vi "sample4(SyncRW X).vi"() -> ()   [LabVIEW 2020]
panel:
  in  "OffsetTime":u32=500
  out "SyncRead Data":cluster{"ID":u8, "Error":u16, "RTTick":u16}[](array[cluster]) {"Error" format="%04x"}
  in  "id3":u8=3 max=253
  in  "id2":u8=2 max=253
  in  "id1":u8=1 max=253
  in  "pos3":i32(knob)
  in  "STOP":bool
  in  "pos2":i32(knob)
  in  "pos1":i32(knob)
  in  "COM":refnum<visa-resource-name> caption="COMポート"
  in  "Baudrate":i32=57600
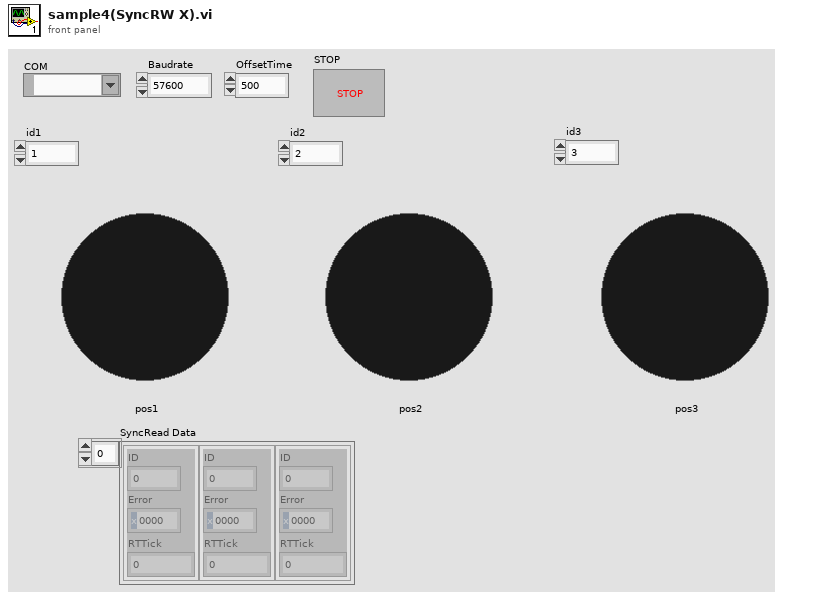
[diagram p1: front panel]
types:
  T1 = cluster{"X Address":u16, "size":u16, cluster{"id3":u8, "array":u8[]}[]}
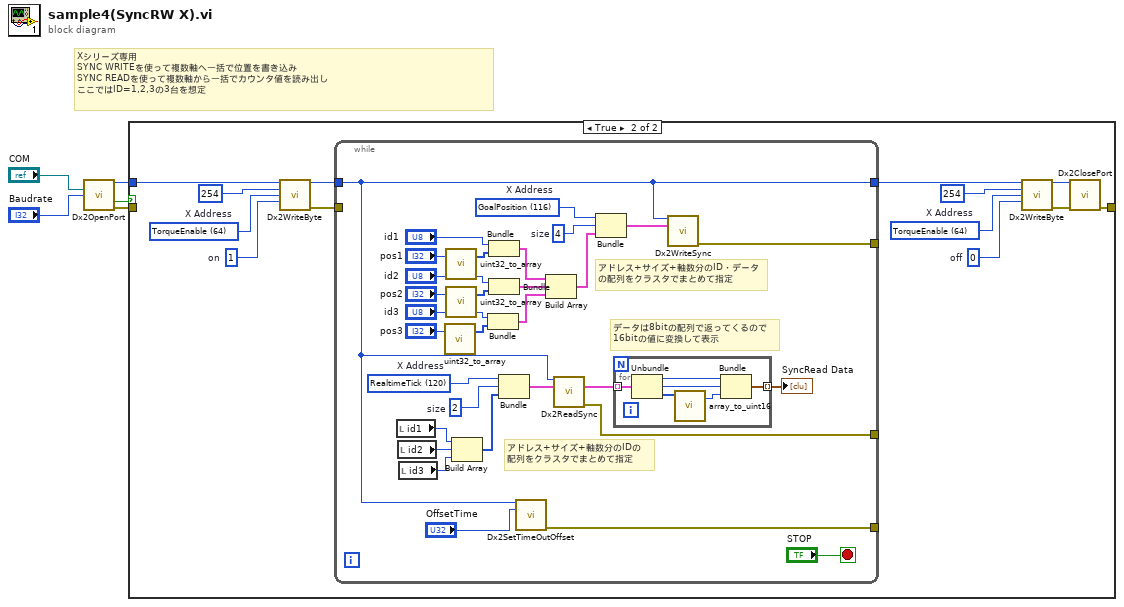
[diagram p0: block diagram]
diagram:
  # "Xシリーズ専用\nSYNC WRITEを使って複数軸へ一括で位置を書き込み\nSYNC READを使って複数軸から一括でカウンタ値を読み出し\nここではID=1,2,3の3台を想定"
  n1 = call "Dx2OpenPort.vi"("port"="COM", "baudrate"="Baudrate") -> ("dvid"=w5:u32, "成功"=w2:bool, "エラー出力"=w1:errorcluster)  [unwired: 11 in]
  n2 = case shown="TRUE" w2 {
    tunnel: w5 -> [_ w17]
    tunnel: w1 -> [_ _]
    tunnel: [_ w13] -> _
    frame False {
    }
    frame True {
      w7 = u16 64 items=["ModelNo"=0, "ModelInfo"=2, "VersionOfFirmware"=6, "ID"=7, "Baudrate"=8, "ReturnDelayTime"=9, "OperationMode"=11, "ProtocolVersion"=13, "HormingOffset"=20, "MovingThreshold"=24, "TemperatureLimit"=31, "MaxVoltageLimit"=32, "MinVoltageLimit"=34, "PWMLimit"=36, "CurrentLimit"=38, "AccelerationLimit"=40, "VelocityLimit"=44, "MaxPositionLimit"=48, "MinPositionLimit"=52, "Shutdown"=63, "TorqueEnable"=64, "LED"=65, "StatusReturnLevel"=68, "RegistedInstruction"=69, "HardwareErrorStatus"=70, "VelocityIGain"=76, "VelocityPGain"=78, "VelocityDGain"=80, "PositionIGain"=82, "PositionPGain"=84, "FeedForward2ndGain"=88, "FeedForward1stGain"=90, "GoalPWM"=100, "GoalCurrent"=102, "GoalVelocity"=104, "ProfileAcceleration"=108, "ProfileVelocity"=112, "GoalPosition"=116, "RealtimeTick"=120, "Moving"=122, "MovingStatus"=123, "PresentPWM"=124, "PresentCurrent"=126, "Presentvelocity"=128, "PresentPosition"=132, "VelocityTrajectory"=136, "PositionTrajectory"=140, "PresentIInputVoltage"=144, "PresentTemperature"=146, "Backup Ready"=147]  # X Address
      w6 = u16 64 items=["ModelNo"=0, "ModelInfo"=2, "VersionOfFirmware"=6, "ID"=7, "Baudrate"=8, "ReturnDelayTime"=9, "OperationMode"=11, "ProtocolVersion"=13, "HormingOffset"=20, "MovingThreshold"=24, "TemperatureLimit"=31, "MaxVoltageLimit"=32, "MinVoltageLimit"=34, "PWMLimit"=36, "CurrentLimit"=38, "AccelerationLimit"=40, "VelocityLimit"=44, "MaxPositionLimit"=48, "MinPositionLimit"=52, "Shutdown"=63, "TorqueEnable"=64, "LED"=65, "StatusReturnLevel"=68, "RegistedInstruction"=69, "HardwareErrorStatus"=70, "VelocityIGain"=76, "VelocityPGain"=78, "VelocityDGain"=80, "PositionIGain"=82, "PositionPGain"=84, "FeedForward2ndGain"=88, "FeedForward1stGain"=90, "GoalPWM"=100, "GoalCurrent"=102, "GoalVelocity"=104, "ProfileAcceleration"=108, "ProfileVelocity"=112, "GoalPosition"=116, "RealtimeTick"=120, "Moving"=122, "MovingStatus"=123, "PresentPWM"=124, "PresentCurrent"=126, "Presentvelocity"=128, "PresentPosition"=132, "VelocityTrajectory"=136, "PositionTrajectory"=140, "PresentIInputVoltage"=144, "PresentTemperature"=146, "Backup Ready"=147]  # X Address
      w11 = u8 0  # off
      w18 = u8 1  # on
      n3 = call "Dx2WriteByte.vi"("dvid in"=w17, "id"=u8 254, "address"=w6, "data in"=w18) -> ("dvid out"=w15:u32, "エラー出力"=w14:errorcluster)  [unwired: 9 in, 1 out]
      n4 = while {
        tunnel: [w48] -> _
        tunnel: [w46] -> _
        tunnel: w15 -> [w23]
        tunnel: w14 -> [_]
        tunnel: [w24] -> _
        tunnel: [w23] -> w9
        stop <- "STOP" stop-if-true
        w19 = u16 120 items=["ModelNo"=0, "ModelInfo"=2, "VersionOfFirmware"=6, "ID"=7, "Baudrate"=8, "ReturnDelayTime"=9, "OperationMode"=11, "ProtocolVersion"=13, "HormingOffset"=20, "MovingThreshold"=24, "TemperatureLimit"=31, "MaxVoltageLimit"=32, "MinVoltageLimit"=34, "PWMLimit"=36, "CurrentLimit"=38, "AccelerationLimit"=40, "VelocityLimit"=44, "MaxPositionLimit"=48, "MinPositionLimit"=52, "Shutdown"=63, "TorqueEnable"=64, "LED"=65, "StatusReturnLevel"=68, "RegistedInstruction"=69, "HardwareErrorStatus"=70, "VelocityIGain"=76, "VelocityPGain"=78, "VelocityDGain"=80, "PositionIGain"=82, "PositionPGain"=84, "FeedForward2ndGain"=88, "FeedForward1stGain"=90, "GoalPWM"=100, "GoalCurrent"=102, "GoalVelocity"=104, "ProfileAcceleration"=108, "ProfileVelocity"=112, "GoalPosition"=116, "RealtimeTick"=120, "Moving"=122, "MovingStatus"=123, "PresentPWM"=124, "PresentCurrent"=126, "Presentvelocity"=128, "PresentPosition"=132, "VelocityTrajectory"=136, "PositionTrajectory"=140, "PresentIInputVoltage"=144, "PresentTemperature"=146, "Backup Ready"=147]  # X Address
        w20 = u16 116 items=["ModelNo"=0, "ModelInfo"=2, "VersionOfFirmware"=6, "ID"=7, "Baudrate"=8, "ReturnDelayTime"=9, "OperationMode"=11, "ProtocolVersion"=13, "HormingOffset"=20, "MovingThreshold"=24, "TemperatureLimit"=31, "MaxVoltageLimit"=32, "MinVoltageLimit"=34, "PWMLimit"=36, "CurrentLimit"=38, "AccelerationLimit"=40, "VelocityLimit"=44, "MaxPositionLimit"=48, "MinPositionLimit"=52, "Shutdown"=63, "TorqueEnable"=64, "LED"=65, "StatusReturnLevel"=68, "RegistedInstruction"=69, "HardwareErrorStatus"=70, "VelocityIGain"=76, "VelocityPGain"=78, "VelocityDGain"=80, "PositionIGain"=82, "PositionPGain"=84, "FeedForward2ndGain"=88, "FeedForward1stGain"=90, "GoalPWM"=100, "GoalCurrent"=102, "GoalVelocity"=104, "ProfileAcceleration"=108, "ProfileVelocity"=112, "GoalPosition"=116, "RealtimeTick"=120, "Moving"=122, "MovingStatus"=123, "PresentPWM"=124, "PresentCurrent"=126, "Presentvelocity"=128, "PresentPosition"=132, "VelocityTrajectory"=136, "PositionTrajectory"=140, "PresentIInputVoltage"=144, "PresentTemperature"=146, "Backup Ready"=147]  # X Address
        w36 = u16 4  # size
        w42 = u16 2  # size
        # "データは8bitの配列で返ってくるので\n16bitの値に変換して表示"
        # "アドレス+サイズ+軸数分のIDの\n配列をクラスタでまとめて指定"
        # "アドレス+サイズ+軸数分のID・データ\nの配列をクラスタでまとめて指定"
        n5 = local read "id1"() -> (w45:u8)
        n6 = local read "id2"() -> (w44:u8)
        n7 = local read "id3"() -> (w43:u8)
        n8 = call "uint32_to_array.vi"("uint32"="pos3") -> ("array"=w33:u8[])  [unwired: 2 in]
        n9 = call "uint32_to_array.vi"("uint32"="pos1") -> ("array"=w34:u8[])  [unwired: 2 in]
        n10 = call "uint32_to_array.vi"("uint32"="pos2") -> ("array"=w32:u8[])  [unwired: 2 in]
        n11 = Build Array(w45, w44, w43) -> (w41:u8[])
        n12 = Bundle("id3"="id3", "array"=w33) -> (w28:cluster{"id3":u8, "array":u8[]})  [unwired: 1 in]
        n13 = Bundle("id1"="id1", "array"=w34) -> (w27:cluster{"id1":u8, "array":u8[]})  [unwired: 1 in]
        n14 = Bundle("id2"="id2", "array"=w32) -> (w29:cluster{"id2":u8, "array":u8[]})  [unwired: 1 in]
        n15 = Bundle("X Address"=w19, "size"=w42, w41) -> (w40:cluster{"X Address":u16, "size":u16, u8[]})  [unwired: 1 in]
        n16 = call "Dx2SetTimeOutOffset.vi"("dvid in"=w23, "OffsetTime"="OffsetTime") -> ("エラー出力"=w46:errorcluster)  [unwired: 12 in, 1 out]
        n17 = Build Array(w27, w29, w28) -> (w26:cluster{"id3":u8, "array":u8[]}[])
        n18 = call "Dx2ReadSync.vi"("dvid in"=w23, "Param"=w40) -> ("data out"=w22:cluster{"ID":u8, "Error":u16, "Data":u8[]}[], "エラー出力"=w48:errorcluster)  [unwired: 10 in, 2 out]
        n19 = Bundle("X Address"=w20, "size"=w36, w26) -> (w25:T1)  [unwired: 1 in]
        n20 = for {
          tunnel: w22 -> [w55] mode=indexing
          tunnel: [w50] -> w21 mode=indexing
          n21 = Unbundle(w55) -> ("ID"=w51:u8, "Error"=w52:u16, "Data"=w54:u8[])
          n22 = call "array_to_uint16.vi"("array"=w54) -> ("uint16"=w53:u16)  [unwired: 6 in]
          n23 = Bundle("ID"=w51, "Error"=w52, "uint16"=w53) -> (w50:cluster{"ID":u8, "Error":u16, "uint16":u16})  [unwired: 1 in]
        }
        "SyncRead Data" <- w21
        n24 = call "Dx2WriteSync.vi"("dvid in"=w23, "data in"=w25) -> ("エラー出力"=w24:errorcluster)  [unwired: 11 in, 2 out]
      }
      n25 = call "Dx2WriteByte.vi"("dvid in"=w9, "id"=u8 254, "address"=w7, "data in"=w11) -> ("dvid out"=w8:u32, "エラー出力"=w10:errorcluster)  [unwired: 9 in, 1 out]
      n26 = call "Dx2ClosePort.vi"("dvid"=w8, "エラー入力"=w10) -> ("エラー出力"=w13:errorcluster)  [unwired: 12 in, 1 out]
    }
  }
